vi "鼠标单击棋子.vi"(0 "按钮":bool[][](array[boolean])) -> (1 "X":i32, 2 "Y":i32, 3 "是否单击":bool)   [LabVIEW 2017]
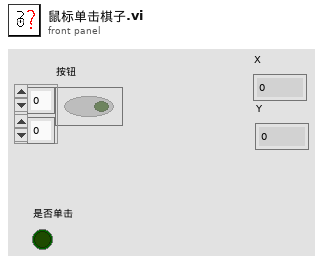
[diagram p1: front panel]
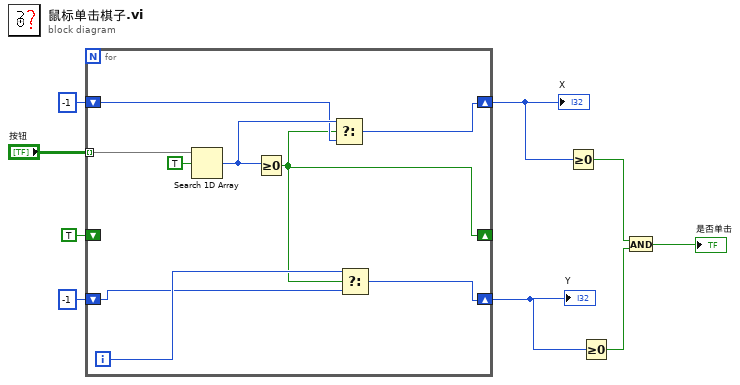
[diagram p0: block diagram]
diagram:
  n1 = for {
    tunnel: "按钮" -> [w18] mode=indexing
    shift-right: [w12] -> w5
    shift-left: -1 ("index of element") -> [w11]
    shift-right: [w13] -> w4
    shift-left: -1 -> [w14]
    shift-right: [w10] -> _
    shift-left: TRUE -> [_]
    i -> [w16]
    n2 = Search 1D Array(1D array=w18, element=TRUE ("元素")) -> (index of element=w15:i32)  [unwired: 1 in]
    n3 = Greater Or Equal To 0?(x=w15) -> (x >= 0?=w10:bool)
    n4 = Select(t=w15, s=w10, f=w11) -> (s? t:f=w12:i32)
    n5 = Select(t=w16, s=w10, f=w14) -> (s? t:f=w13:i32)
  }
  "X" <- w5
  "Y" <- w4
  n6 = Greater Or Equal To 0?(x=w5) -> (x >= 0?=w3:bool)
  n7 = Greater Or Equal To 0?(x=w4) -> (x >= 0?=w2:bool)
  n8 = And(x=w3, y=w2) -> (x .and. y?=→"是否单击":bool)
